vi "LoadController.vi"(8 "error in (no error)":errorcluster, 10 "Actor In":refnum<class "Actor.lvclass">, 11 "Device in":refnum<class "Device.lvclass">) -> (0 "error out":errorcluster, 3 "Device out":refnum<class "Device.lvclass">)   [LabVIEW 2020, in "Device.lvlib" / "Device.lvclass"]
uses:
  Device.lvclass
  C:/Program Files/National Instruments/LabVIEW 2020/vi.lib/ActorFramework/Actor/Actor.lvclass
  <vilib>/ActorFramework/Actor/Actor.lvclass
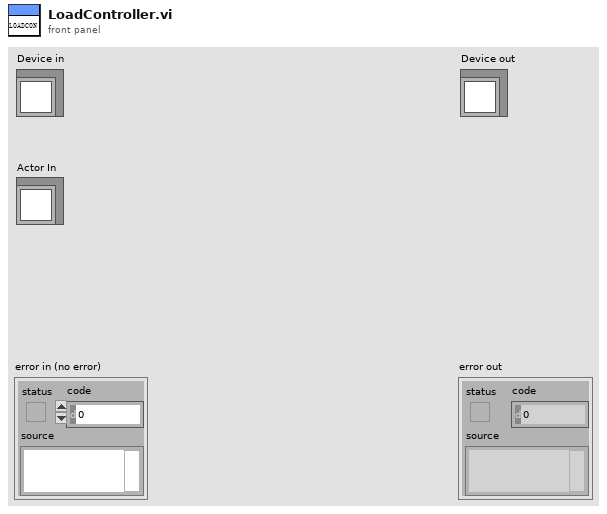
[diagram p1: front panel]
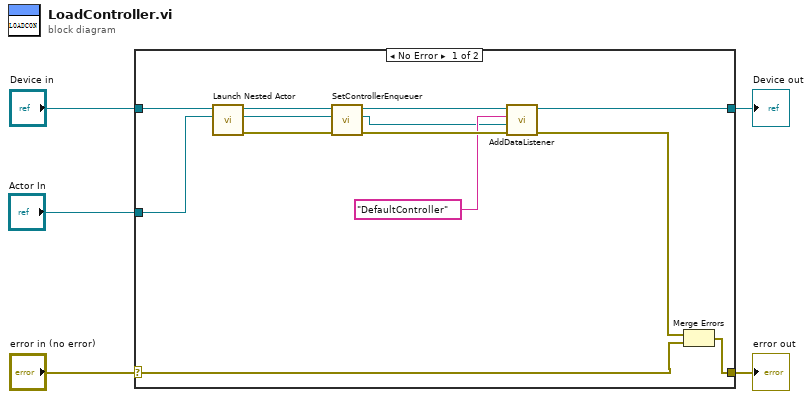
[diagram p0: block diagram]
diagram:
  n1 = case shown="No Error" "error in (no error)" {
    selector: "error in (no error)" -> [w13 w20]
    tunnel: [w12 w20] -> w4
    tunnel: [w8 w19] -> w2
    tunnel: "Device in" -> [w18 w19]
    tunnel: "Actor In" -> [w17 _]
    frame No Error {
      n2 = call <vilib>:"Launch Nested Actor.vi"("Nested Actor"=w17, "Caller Actor in"=w18) -> ("error out"=w14:errorcluster, "Nested Actor's Enqueuer"=w15:refnum<class "Message Enqueuer.lvclass">, "Caller Actor out"=w16:refnum<class "Device.lvclass">)  [unwired: 7 in]
      n3 = call-dynamic "SetControllerEnqueuer.vi"("error in (no error)"=w14, "Controller Enqueuer"=w15, "Device in"=w16) -> ("error out"=w11:errorcluster, "Controller Enqueue Out"=w6:refnum<class "Message Enqueuer.lvclass">, "Device out"=w9:refnum<class "Device.lvclass">)  [unwired: 6 in]
      n4 = call-dynamic "AddDataListener.vi"("error in (no error)"=w11, "Listener In"=w6, "Label"="DefaultController", "Device in"=w9) -> ("error out"=w10:errorcluster, "Device out"=w8:refnum<class "Device.lvclass">)  [unwired: 6 in]
      n5 = Merge Errors(w10, w13) -> (w12:errorcluster)
    }
    frame Error {
    }
  }
  "error out" <- w4
  "Device out" <- w2
